vi "Callback Change Channel Name.vi"(6 "Variant":variant, 8 "error in (no error)":errorcluster, 9 "Old Values":string[][](array[string]), 10 "object ref in":T1, 11 "Table Change":T2) -> (0 "error out":errorcluster)   [LabVIEW 2015, in "Sequencer Module editor node.lvclass"]
doc: "This VI gets called automatically when changes are made to the 'Name' column of the table and must handle changes appropriately. Register this callback using the appropriate 'Define Column' VI from the Table API."
uses:
  Sequencer Module editor node.lvclass
  <vilib>/NI/DCAF/Tag Editor Core/Table API/Table Manager/Cell Change.ctl
  <vilib>/NI/DCAF/Tag Editor Core/Table API/Table Manager/object ref.ctl
  <vilib>/NI/DCAF/Tag Editor Core/Configuration Editor/Classes/Engine Parent/Engine Parent Editor Node.lvclass
  <vilib>/NI/DCAF/Tag Editor Core/Configuration Editor/Classes/Module editor node/module editor node.lvclass
  module/configuration/Sequencer Module configuration.lvclass
  <vilib>/NI/Tag Bus/tag/tag descriptor.lvclass
  <vilib>/NI/Configuration Framework/serializable configuration/NISE_CEF_serializable configuration.lvclass
  <vilib>/NI/Module Execution Interface/Engine Configuration/engine configuration.lvclass
  <vilib>/NI/DCAF/Tag Editor Core/Table API/Table Manager.lvlib
  <vilib>/NI/DCAF/Tag Editor Core/Table API/Table Manager/Table Manager.lvclass
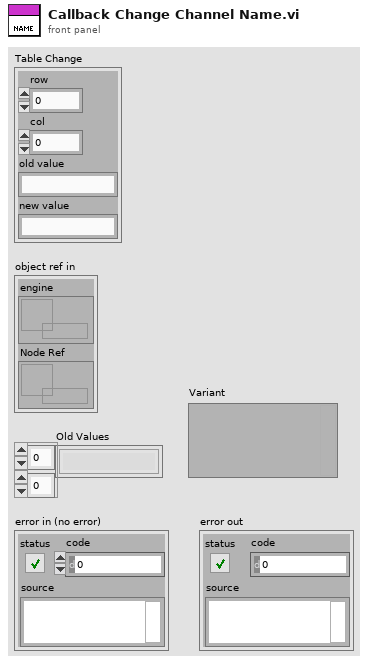
[diagram p1: front panel]
types:
  T1 = typedef "Table Manager.lvclass/object ref.ctl" = cluster{"engine":refnum<data-value>, "Node Ref":refnum<data-value>}
  T2 = typedef "Table Manager.lvlib/Cell Change.ctl" = cluster{"row":i32, "col":i32, "old value":string, "new value":string}
  T3 = typedef "Sequencer Module configuration.lvclass/Line.ctl" = cluster{"Sequence":refnum<class "Sequence Config.lvclass">}
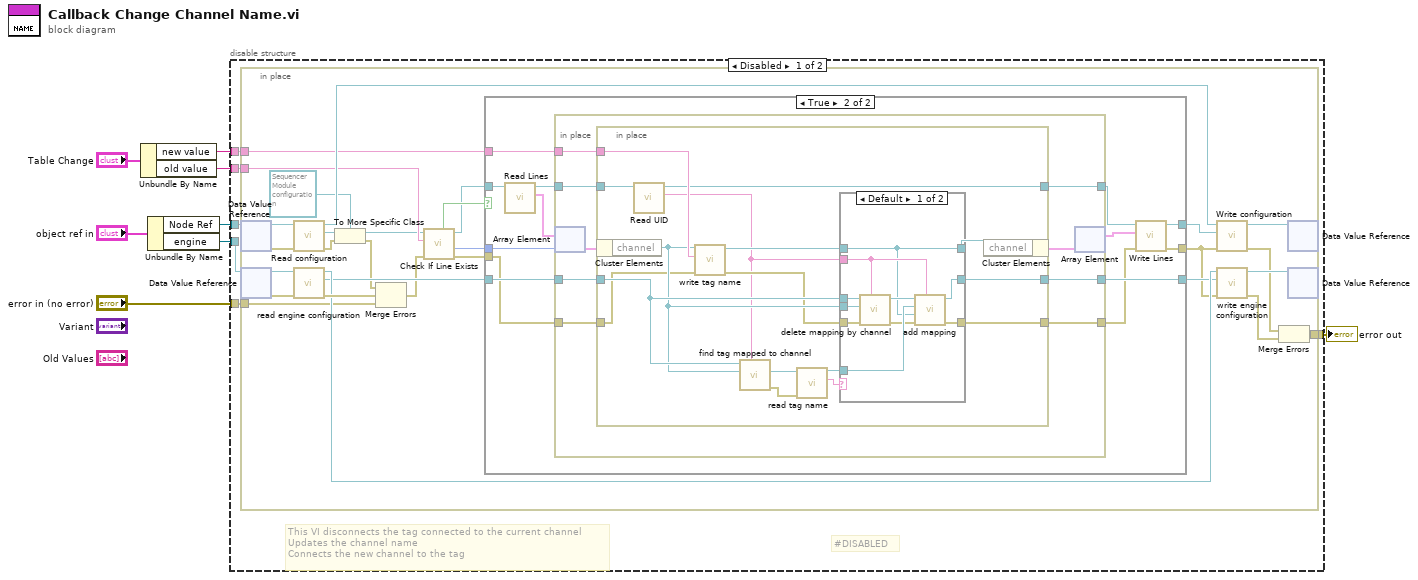
[diagram p0: block diagram]
diagram:
  n1 = Unbundle By Name("Table Change") -> ("new value"=w1:string, "old value"=w2:string)
  n2 = Unbundle By Name("object ref in") -> ("Node Ref"=w5:refnum<data-value>, "engine"=w4:refnum<data-value>)
  n3 = disable-structure shown="Disabled" {
    disable-tunnel: [w14 _] -> w8
    disable-tunnel: "error in (no error)" -> [w13 _]
    disable-tunnel: w5 -> [w12 _]
    disable-tunnel: w4 -> [w11 _]
    disable-tunnel: w2 -> [w10 _]
    disable-tunnel: w1 -> [w9 _]
    frame Disabled {
      # "#DISABLED"
      # "This VI disconnects the tag connected to the current channel\nUpdates the channel name\nConnects the new channel to the tag"
      n4 = in-place {
        in-place-border: [w35] -> w14
        in-place-border: w13 -> [w31]
        in-place-border: w10 -> [w29]
        in-place-border: w9 -> [w26]
        n5 = in-place-dvr #1(w12) -> (w24:refnum<class "module editor node.lvclass">, w34:errorcluster)
        n6 = in-place-dvr #2(w11) -> (w42:refnum<class "Engine Parent Editor Node.lvclass">, w43:errorcluster)
        n7 = call-dynamic "Read configuration.vi"("error in"=w34, "NISE_CEF_serializable node in"=w24) -> ("error out"=w16:errorcluster, "configuration"=w32:refnum<class "NISE_CEF_serializable configuration.lvclass">, "NISE_CEF_serializable node out"=w33:refnum<class "module editor node.lvclass">)  [unwired: 7 in]
        n8 = call <vilib>:"read engine configuration.vi"("error in"=w43, "Engine Parent Editor Node in"=w42) -> ("error out"=w39:errorcluster, "engine configuration"=w21:refnum<class "engine configuration.lvclass">, "Engine Parent Editor Node out"=w38:refnum<class "Engine Parent Editor Node.lvclass">)  [unwired: 7 in]
        n9 = To More Specific Class(target class=refnum<class "Sequencer Module configuration.lvclass"> refnum ("tag bus configurable plugin module configuration"), reference=w32, error in=w16) -> (specific class reference=w23:refnum<class "Sequencer Module configuration.lvclass">, error out=w15:errorcluster)
        n10 = Merge Errors(w15, w39, w31) -> (w19:errorcluster)
        n11 = call-dynamic "Check If Line Exists.vi"("error in"=w19, "Name to Locate"=w29, "Sequencer Module configuration in"=w23) -> ("error out"=w20:errorcluster, "Index"=w27:i32, "Sequencer Module configuration out"=w18:refnum<class "Sequencer Module configuration.lvclass">, "Found?"=w25:bool)  [unwired: 4 in, 1 out]
        n12 = case shown="True" w25 {
          tunnel: [w46 w59] -> w28
          tunnel: w18 -> [w46 w58]
          tunnel: w27 -> [_ w55]
          tunnel: w26 -> [_ w54]
          tunnel: w21 -> [w45 w53]
          tunnel: [w45 w52] -> w22
          tunnel: [w44 w51] -> w17
          tunnel: w20 -> [w44 w49]
          frame False {
          }
          frame True {
            n13 = call "Read Lines.vi"("Sequencer Module configuration in"=w58) -> ("Lines"=w57:T3[], "Sequencer Module configuration out"=w48:refnum<class "Sequencer Module configuration.lvclass">)  [unwired: 8 in, 1 out]
            n14 = in-place {
              in-place-border: w54 -> [w66]
              in-place-border: w53 -> [w65]
              in-place-border: [w64] -> w52
              in-place-border: [w63] -> w50
              in-place-border: w49 -> [w62]
              in-place-border: w48 -> [w61]
              in-place-border: [w60] -> w47
              n15 = in-place-array #3(w57, w55) -> (w68:T3)
              n16 = in-place {
                in-place-border: w66 -> [w84]
                in-place-border: w65 -> [w82]
                in-place-border: [w83] -> w64
                in-place-border: [w74] -> w63
                in-place-border: w62 -> [w76]
                in-place-border: w61 -> [w72]
                in-place-border: [w71] -> w60
                n17 = in-place-cluster #4(w68) -> ("channel"=w81:refnum<class "TBM channel.lvclass">)
                n18 = call <vilib>:"Read UID.vi"("configuration in"=w72) -> ("instance id"=w73:string, "configuration out"=w71:refnum<class "Sequencer Module configuration.lvclass">)  [unwired: 8 in, 1 out]
                n19 = call <vilib>:"write tag name.vi"("error in"=w76, "name"=w84, "system tag in"=w81) -> ("error out"=w75:errorcluster, "system tag out"=w77:refnum<class "TBM channel.lvclass">)  [unwired: 7 in]
                n20 = call <vilib>:"find tag mapped to channel.vi"("owner"=w73, "channel"=w81, "engine configuration in"=w82) -> ("error out"=w69:errorcluster, "tag"=w80:refnum<class "tag descriptor.lvclass">)  [unwired: 6 in, 1 out]
                n21 = call <vilib>:"read tag name.vi"("error in"=w69, "system tag in"=w80) -> ("name"=w79:string, "system tag out"=w78:refnum<class "tag descriptor.lvclass">)  [unwired: 7 in, 1 out]
                n22 = case shown="Default" w79 {
                  tunnel: [w93 w97] -> w83
                  tunnel: w82 -> [w92 w97]
                  tunnel: w73 -> [w91 _]
                  tunnel: w81 -> [w90 _]
                  tunnel: w78 -> [w89 _]
                  tunnel: w77 -> [w85 w95]
                  tunnel: [w87 w96] -> w74
                  tunnel: w75 -> [w86 w96]
                  tunnel: [w85 w95] -> w70
                  frame Default {
                    n23 = call <vilib>:"delete mapping by channel.vi"("owner ID"=w91, "error in"=w86, "channel"=w90, "engine configuration in"=w92) -> ("error out"=w88:errorcluster, "engine configuration out"=w94:refnum<class "engine configuration.lvclass">)  [unwired: 6 in]
                    n24 = call-dynamic "add mapping.vi"("owner ID"=w91, "error in"=w88, "channel"=w85, "tag descriptor"=w89, "engine configuration"=w94) -> ("error out"=w87:errorcluster, "engine configuration out"=w93:refnum<class "engine configuration.lvclass">)  [unwired: 5 in]
                  }
                  frame "" {
                  }
                }
                n25 = in-place-cluster #4("channel"=w70) -> (w67:T3)
              }
              n26 = in-place-array #3(w67) -> (w56:T3[])  [unwired: 1 out]
            }
            n27 = call "Write Lines.vi"("error in (no error)"=w50, "Lines"=w56, "Sequencer Module configuration in"=w47) -> ("error out"=w51:errorcluster, "Sequencer Module configuration out"=w59:refnum<class "Sequencer Module configuration.lvclass">)  [unwired: 7 in]
          }
        }
        n28 = call-dynamic "Write configuration.vi"("error in"=w17, "configuration"=w28, "NISE_CEF_serializable node in"=w33) -> ("error out"=w36:errorcluster, "NISE_CEF_serializable node out"=w40:refnum<class "module editor node.lvclass">)  [unwired: 7 in]
        n29 = call <vilib>:"write engine configuration.vi"("error in"=w17, "engine configuration"=w22, "Engine Parent Editor Node in"=w38) -> ("error out"=w37:errorcluster, "Engine Parent Editor Node out"=w41:refnum<class "Engine Parent Editor Node.lvclass">)  [unwired: 7 in]
        n30 = Merge Errors(w36, w37) -> (w35:errorcluster)
        n31 = in-place-dvr #1(w40) -> ()  [unwired: 2 out]
        n32 = in-place-dvr #2(w41) -> ()  [unwired: 2 out]
      }
    }
    frame Enabled {
    }
  }
  "error out" <- w8
